vi "Get Port Widths in Bits.vi"(11 "niInstr AXI4-Stream Writer FXP64x4 v1 FPGA in":refnum<class "niInstr AXI4-Stream Writer FXP64x4 v1 FPGA.lvclass">) -> (2 "port widths":T1, 3 "niInstr AXI4-Stream Writer FXP64x4 v1 FPGA out":refnum<class "niInstr AXI4-Stream Writer FXP64x4 v1 FPGA.lvclass">)   [LabVIEW 2015, in "niInstr AXI4-Stream Writer FXP64x4 v1 FPGA.lvclass"]
uses:
  <instrlib>/_niInstr/CLIP Adapters/v1/FPGA/AXI4-Stream/Writer FXP64x4/niInstr AXI4-Stream Writer FXP64x4 v1 FPGA.lvclass
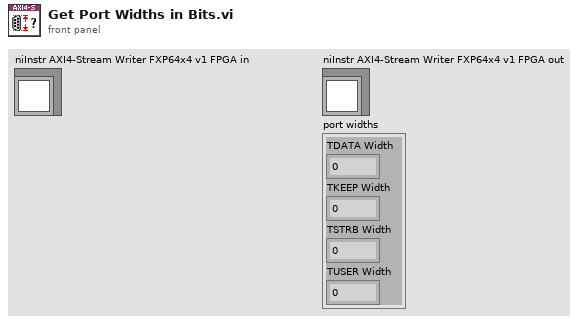
[diagram p1: front panel]
types:
  T1 = cluster{"TDATA Width":i16, "TKEEP Width":i16, "TSTRB Width":i16, "TUSER Width":i16}
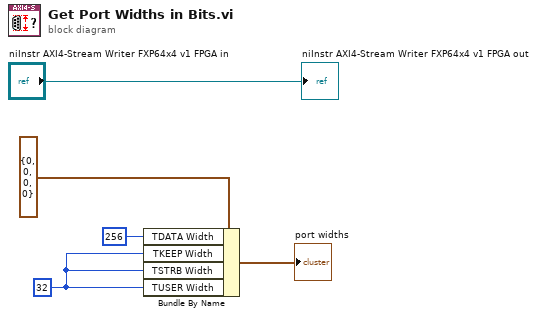
[diagram p0: block diagram]
diagram:
  w4 = i16 32 ("TKEEP Width (Bits)")
  n1 = Bundle By Name(cluster=T1 {"TDATA Width"=0, "TKEEP Width"=0, "TSTRB Width"=0, "TUSER Width"=0} ("Port Widths"), "TDATA Width"=i16 256 ("TDATA Width (Bits)"), "TKEEP Width"=w4, "TSTRB Width"=w4, "TUSER Width"=w4) -> (→"port widths":T1)
  "niInstr AXI4-Stream Writer FXP64x4 v1 FPGA out" <- "niInstr AXI4-Stream Writer FXP64x4 v1 FPGA in"
